vi "Read Magnetometer Range.vi"(8 "error in (no error)":errorcluster, 11 "LSM9DS1 IMU in":refnum<class "LSM9DS1 IMU.lvclass">) -> (0 "error out":errorcluster, 2 "Magnetometer Range":T1, 3 "LSM9DS1 IMU out":refnum<class "LSM9DS1 IMU.lvclass">)   [LabVIEW 2020, in "LSM9DS1 IMU.lvclass"]
uses:
  LSM9DS1 IMU.lvclass
  Magnetometer Range.ctl
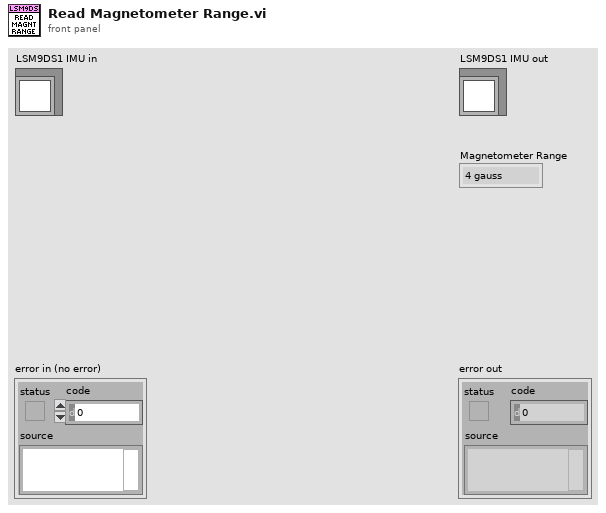
[diagram p1: front panel]
types:
  T1 = typedef "LSM9DS1 IMU.lvclass/Magnetometer Range.ctl" = enum16{"4 gauss", "8 gauss", "12 gauss", "16 gauss"}
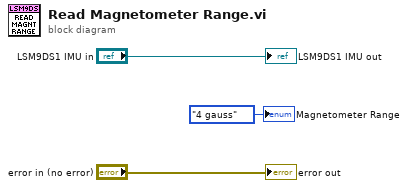
[diagram p0: block diagram]
diagram:
  "error out" <- "error in (no error)"
  "LSM9DS1 IMU out" <- "LSM9DS1 IMU in"
  "Magnetometer Range" <- Magnetometer_Range."4 gauss" ("Magnetometer Range")
